vi "Set Plot Names.vi"(8 "error in (no error)":errorcluster, 10 "Plot Names":string[](array[string]), 11 "Graph Reference":refnum<vi>) -> (0 "error out":errorcluster)   [LabVIEW 2010]
doc: "This VI is used to set the plot names on a Waveform Chart or Waveform Graph."
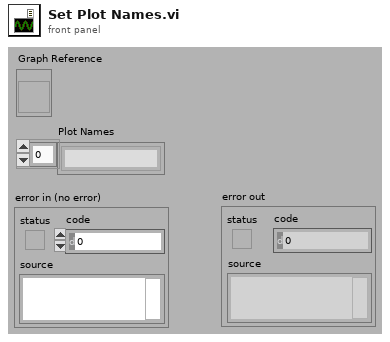
[diagram p1: front panel]
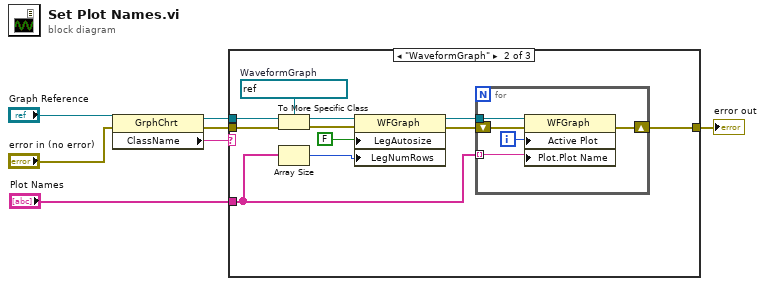
[diagram p0: block diagram]
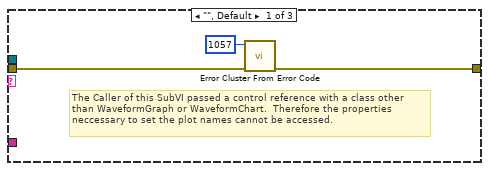
[diagram p2: hidden frame]
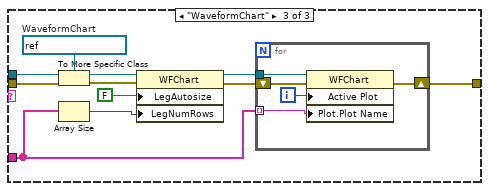
[diagram p3: hidden frame]
diagram:
  n1 = property class="GrphChrt"(reference="Graph Reference", error in="error in (no error)") -> (reference out=w4:refnum<vi>, error out=w5:errorcluster, "ClassName"=w6:string)
  n2 = case shown="\"WaveformGraph\"" w6 {
    tunnel: w5 -> [w9 w15 w31]
    tunnel: w4 -> [_ w16 w32]
    tunnel: "Plot Names" -> [_ w11 w27]
    tunnel: [w8 w13 w29] -> w1
    frame "", Default {
      # "The Caller of this SubVI passed a control reference with a class other\nthan WaveformGraph or WaveformChart.  Therefore the properties\nneccessary to set the plot names cannot be accessed."
      n3 = call <vilib>:"Error Cluster From Error Code.vi"("error in (no error)"=w9, "error code (0)"=1057) -> ("error out"=w8:errorcluster)  [unwired: 7 in]
    }
    frame "WaveformGraph" {
      w21 = refnum<vi> refnum  # WaveformGraph
      n4 = To More Specific Class(target class=w21, reference=w16, error in=w15) -> (specific class reference=w19:refnum<vi>, error out=w20:errorcluster)
      n5 = Array Size(array=w11) -> (size(s)=w12:i32)
      n6 = property class="WFGraph"(reference=w19, error in=w20, "LegAutosize"=FALSE ("Legend:Autosize"), "LegNumRows"=w12) -> (reference out=w17:refnum<vi>, error out=w14:errorcluster)
      n7 = for {
        tunnel: w17 -> [w26]
        shift-right: [w24] -> w13
        shift-left: w14 -> [w25]
        tunnel: w11 -> [w22] mode=indexing
        i -> [w23]
        n8 = property class="WFGraph"(reference=w26, error in=w25, "Active Plot"=w23, "Plot.Plot Name"=w22) -> (error out=w24:errorcluster)  [unwired: 1 out]
      }
    }
    frame "WaveformChart" {
      w37 = refnum<vi> refnum  # WaveformChart
      n9 = To More Specific Class(target class=w37, reference=w32, error in=w31) -> (specific class reference=w35:refnum<vi>, error out=w36:errorcluster)
      n10 = Array Size(array=w27) -> (size(s)=w28:i32)
      n11 = property class="WFChart"(reference=w35, error in=w36, "LegAutosize"=FALSE ("Legend:Autosize"), "LegNumRows"=w28) -> (reference out=w33:refnum<vi>, error out=w30:errorcluster)
      n12 = for {
        tunnel: w33 -> [w42]
        shift-right: [w40] -> w29
        shift-left: w30 -> [w41]
        tunnel: w27 -> [w38] mode=indexing
        i -> [w39]
        n13 = property class="WFChart"(reference=w42, error in=w41, "Active Plot"=w39, "Plot.Plot Name"=w38) -> (error out=w40:errorcluster)  [unwired: 1 out]
      }
    }
  }
  "error out" <- w1
